vi "Get Currents & Ranges.vi"(0 "CS.lvclass in":refnum<class "CS.lvclass">, 5 "error in (no error)":errorcluster) -> (14 "CS.lvclass out":refnum<class "CS.lvclass">, 15 "I0":cluster{"Value":dbl, "Range":dbl}, 16 "I1":cluster{"Value":dbl, "Range":dbl}, 17 "I2":cluster{"Value":dbl, "Range":dbl}, 18 "I3":cluster{"Value":dbl, "Range":dbl}, 19 "error out":errorcluster)   [LabVIEW 2013, in "CS.lvclass"]
uses:
  Lib.llb/CS.lvclass
  Lib.llb/CS.lvclass/CS.ctl
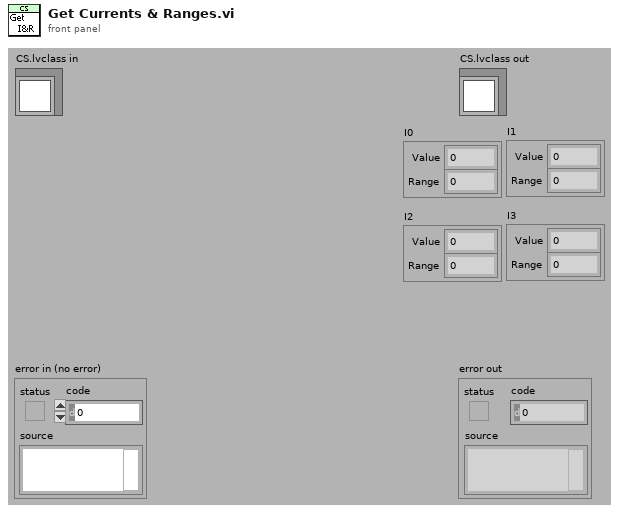
[diagram p1: front panel]
types:
  T1 = cluster{"Range":u8, "Current":dbl, "Current (string)":string, "On?":bool, "G?":bool, "I?":bool, "Err?":bool}
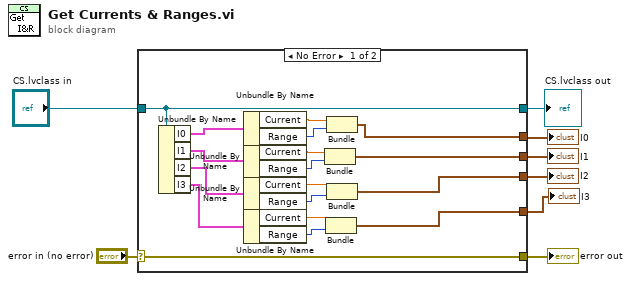
[diagram p0: block diagram]
diagram:
  n1 = case shown="No Error" "error in (no error)" {
    selector: "error in (no error)" -> [w26 w27]
    tunnel: [w26 w27] -> w7
    tunnel: [w25 w28] -> w5
    tunnel: "CS.lvclass in" -> [w25 w28]
    tunnel: [w12 _] -> w4
    tunnel: [w11 _] -> w3
    tunnel: [w10 _] -> w2
    tunnel: [w9 _] -> w1
    frame No Error {
      n2 = Unbundle By Name(w25) -> ("I0"=w24:T1, "I1"=w22:T1, "I2"=w21:T1, "I3"=w23:T1)
      n3 = Unbundle By Name(w24) -> ("Current"=w20:dbl, "Range"=w19:u8)
      n4 = Unbundle By Name(w22) -> ("Current"=w14:dbl, "Range"=w13:u8)
      n5 = Unbundle By Name(w21) -> ("Current"=w18:dbl, "Range"=w15:u8)
      n6 = Unbundle By Name(w23) -> ("Current"=w17:dbl, "Range"=w16:u8)
      n7 = Bundle("Current"=w14, "Range"=w13) -> (w11:cluster{"Current":dbl, "Range":u8})  [unwired: 1 in]
      n8 = Bundle("Current"=w17, "Range"=w16) -> (w9:cluster{"Current":dbl, "Range":u8})  [unwired: 1 in]
      n9 = Bundle("Current"=w20, "Range"=w19) -> (w12:cluster{"Current":dbl, "Range":u8})  [unwired: 1 in]
      n10 = Bundle("Current"=w18, "Range"=w15) -> (w10:cluster{"Current":dbl, "Range":u8})  [unwired: 1 in]
    }
    frame Error {
    }
  }
  "error out" <- w7
  "CS.lvclass out" <- w5
  "I0" <- w4
  "I1" <- w3
  "I3" <- w1
  "I2" <- w2
